vi "Log Target.vi"(8 "error in (no error)":errorcluster, 10 "Entry":string, 11 "IStudy Actor in":refnum<class "IStudy Actor.lvclass">) -> (0 "error out":errorcluster, 3 "IStudy Actor out":refnum<class "IStudy Actor.lvclass">)   [LabVIEW 2023, in "IStudy Actor.lvlib" / "IStudy Actor.lvclass"]
uses:
  IStudy Actor.lvclass
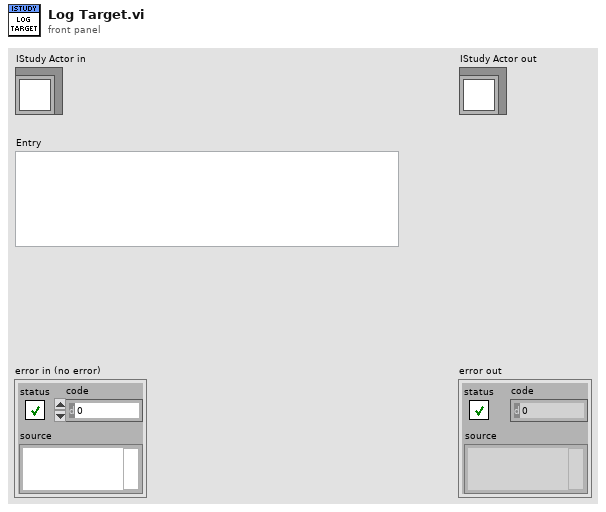
[diagram p1: front panel]
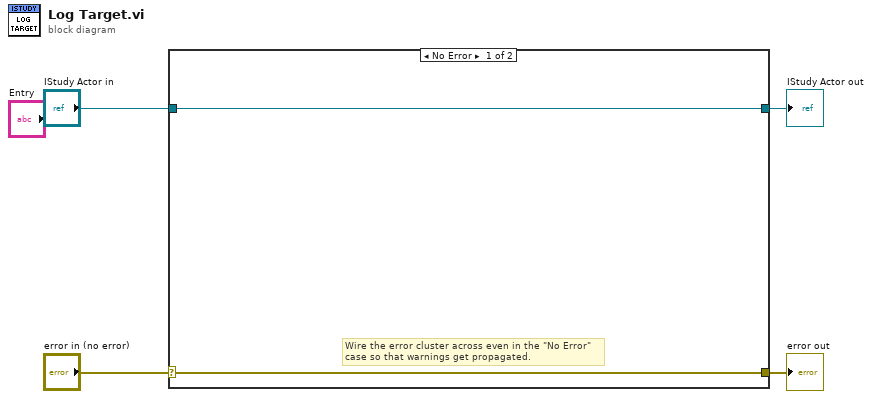
[diagram p0: block diagram]
diagram:
  n1 = case shown="No Error" "error in (no error)" {
    selector: "error in (no error)" -> [w5 w8]
    tunnel: [w5 w8] -> w3
    tunnel: [w6 w7] -> w1
    tunnel: "IStudy Actor in" -> [w6 w7]
    frame No Error {
      # "Wire the error cluster across even in the \"No Error\"\ncase so that warnings get propagated."
    }
    frame Error {
    }
  }
  "error out" <- w3
  "IStudy Actor out" <- w1
